vi "check_db_conn.vi"() -> ()   [LabVIEW 2021]
uses:
  <vilib>/Utility/file.llb/Read Delimited Spreadsheet (string).vi
panel:
  out "Function name in py file":string="db_conn_debugger"
  out "Current VI Path":path
  out "Conn details":string[](array[string])
  out "Postgres Tools Path":path
  out "Conn Path":path
  out "Python version":string
  out "Message Out":string
  in  "error in (no error) py":errorcluster
  out "error out py":errorcluster
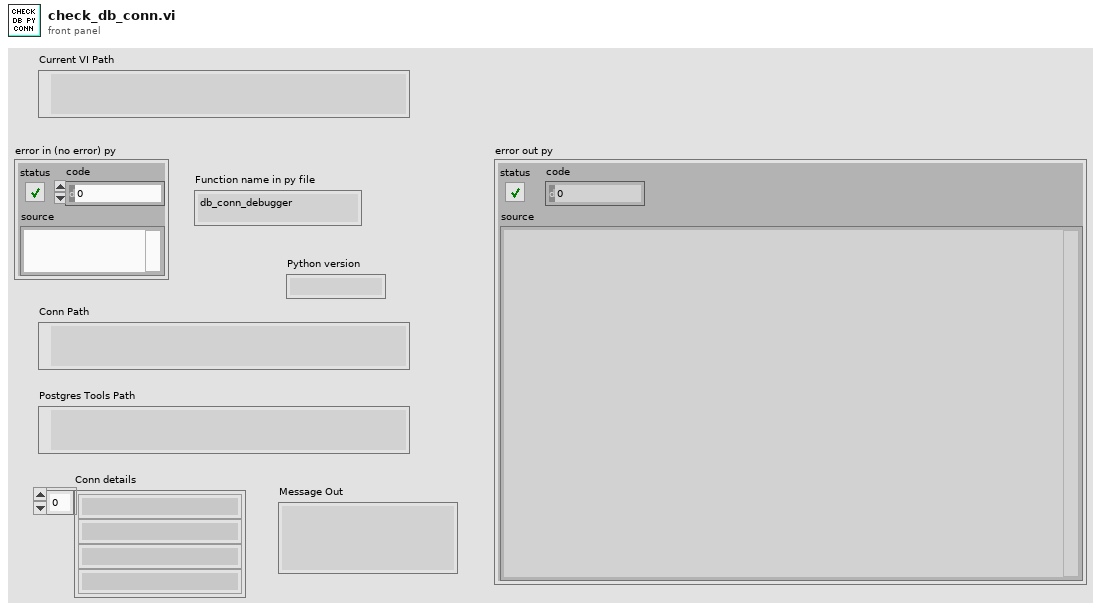
[diagram p1: front panel]
types:
  T1 = typedef "File Paths.ctl" = cluster{"Glue Pattern Folder":path, "Carrier Tray Folder":path, "Pick Up Tool Fixture Folder":path, "Components Folder":path, "Bellows Tool Offset.txt":path, "Pick Up Tool Offset.txt":path, "Dispense Tip Offset.txt":path, "Log Files":path, "Gantry Assembly Map.txt":path, "Syringe and offset map.txt":path, "Controllers Folder":path, "Local dbase config":path}
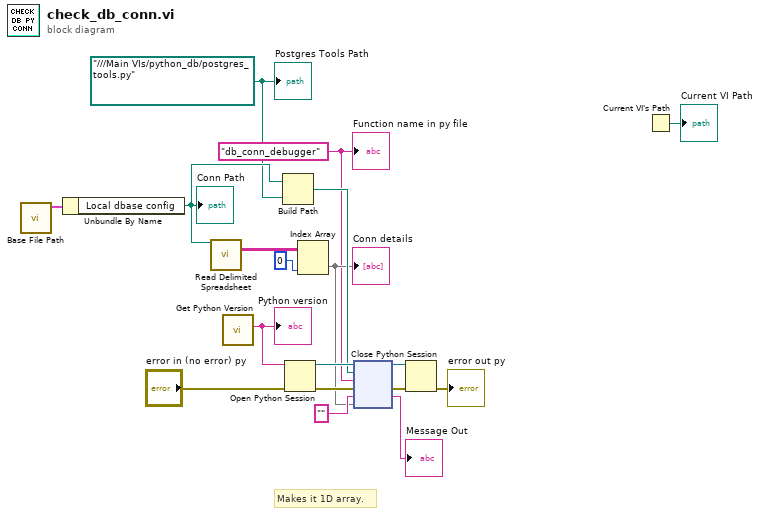
[diagram p0: block diagram]
diagram:
  w1 = "db_conn_debugger" ("function name")
  w4 = path "../../../Main VIs/python_db/postgres_tools.py" ("module path")
  # "Makes it 1D array."
  n1 = call "Base File Path.vi"() -> ("Paths Out"=w12:T1)  [unwired: 11 in]
  n2 = Unbundle By Name(w12) -> ("Local dbase config"=w5:path)
  "Conn Path" <- w5
  n3 = call-poly <vilib>:"Read Delimited Spreadsheet.vi"("file path (dialog if empty)"=w5) -> ("all rows"=w11:string[][])  [unwired: 9 in, 5 out]
  n4 = call "Get Python Version.vi"() -> ("Python Version"=w6:string)  [unwired: 10 in, 1 out]
  "Python version" <- w6
  n5 = Build Path(base path=w5, name or relative path=w4) -> (appended path=w10:path)
  n6 = Open Python Session(python version=w6, 3:"error in (no error) py") -> (session out=w15:refnum<k35>, error out=w17:errorcluster)  [unwired: 1 in]
  n7 = Index Array(array=w11, index (col)=0 ("disabled index (col)")) -> (element=w3:string[])  [unwired: 1 in]
  "Conn details" <- w3
  n8 = node(w15, w10, w1, w17, "", w3) -> (w14:refnum<k35>, w13:errorcluster, →"Message Out":string)  [unwired: 1 in, 2 out]
  n9 = Close Python Session(session in=w14, error in=w13) -> (11:→"error out py":errorcluster)
  n10 = Current VI's Path() -> (path=→"Current VI Path":path)
  "Postgres Tools Path" <- w4
  "Function name in py file" <- w1
